vi "Configure Correction and Temperature.vi"(8 "error in (no error)":errorcluster, 9 "High Temperature Mode (F: Disable)":bool, 10 "System Error Correction (T: Enable)":bool=TRUE, 11 "VISA resource name":refnum<visa-resource-name>) -> (0 "error out":errorcluster, 3 "VISA resource name out":refnum<visa-resource-name>)   [LabVIEW 2012, in "Tektronix TTR500 Series.lvlib"]
doc: "This VI configures correction and temperature."
uses:
  <instrlib>/Tektronix TTR500 Series/Tektronix TTR500 Series.lvlib
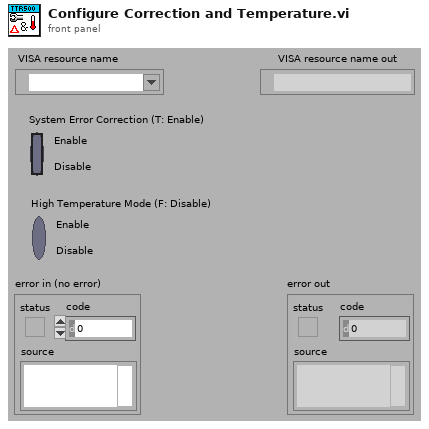
[diagram p1: front panel]
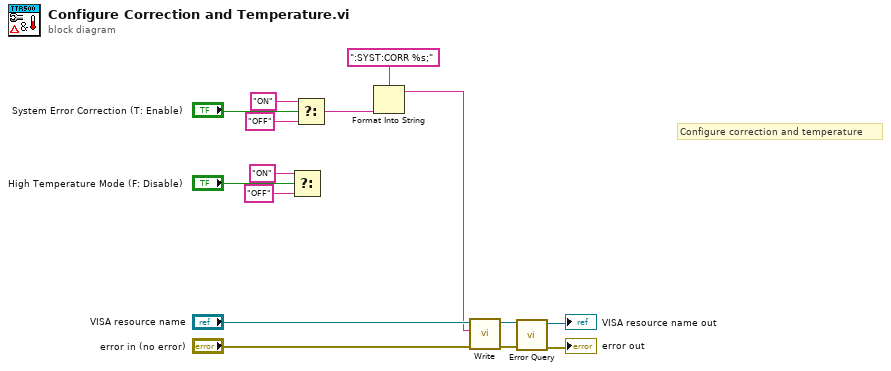
[diagram p0: block diagram]
diagram:
  # "Configure correction and temperature"
  n1 = Select(t="ON", s="High Temperature Mode (F: Disable)", f="OFF") -> ()  [unwired: 1 out]
  n2 = Select(t="ON", s="System Error Correction (T: Enable)", f="OFF") -> (s? t:f=w8:string)
  n3 = Format Into String(format string=":SYST:CORR %s;", w8) -> (resulting string=w2:string)  [unwired: 2 in, 1 out]
  n4 = call <instrlib>:"Write.vi"("error in (no error)"="error in (no error)", "String ()"=w2, "VISA resource name"="VISA resource name") -> ("error out"=w6:errorcluster, "VISA resource name out"=w7:refnum<visa-resource-name>)  [unwired: 6 in, 1 out]
  n5 = call <instrlib>:"Error Query.vi"("error in (no error)"=w6, "VISA resource name"=w7) -> ("error out"=→"error out":errorcluster, "VISA resource name out"=→"VISA resource name out":refnum<visa-resource-name>)  [unwired: 6 in, 2 out]
